vi "20T_Set_Setpoint.vi"(8 "error in (no error)":errorcluster, 10 "20T Control":T1={"Clamp"=TRUE, "Switch Heater"=TRUE, "Go to Zero"=TRUE, "Go to Set"=FALSE, "Go to Hold"=FALSE, "Setpoint (T)"=3.4572, "Rate (T/min)"=0.0, "Set Rate"=FALSE} {"Rate (T/min)" format="%6_5f"; "Setpoint (T)" format="%#4_5f"}, 11 "Mercury Reference In":T2) -> (0 "error out":errorcluster)   [LabVIEW 2016]
uses:
  Equipment/Mercury iXX/Public/Controls/Mercury Reference.ctl
  Equipment/Mercury iXX/Public/Controls/Comms Transport Layer.ctl
  Equipment/Mercury iXX/Private/Controls/Query Dynamic Reference.ctl
  Utility/Monitor Communication/Gustav/20T_Control.ctl
  Equipment/Mercury iXX/Public/Libraries/Magnet/Open/Open Magnet Device.vi
  Equipment/Mercury iXX/Mercury iXX.lvlib
  Equipment/Mercury iXX/Public/Libraries/Magnet.lvlib
panel:
  # "20 T"
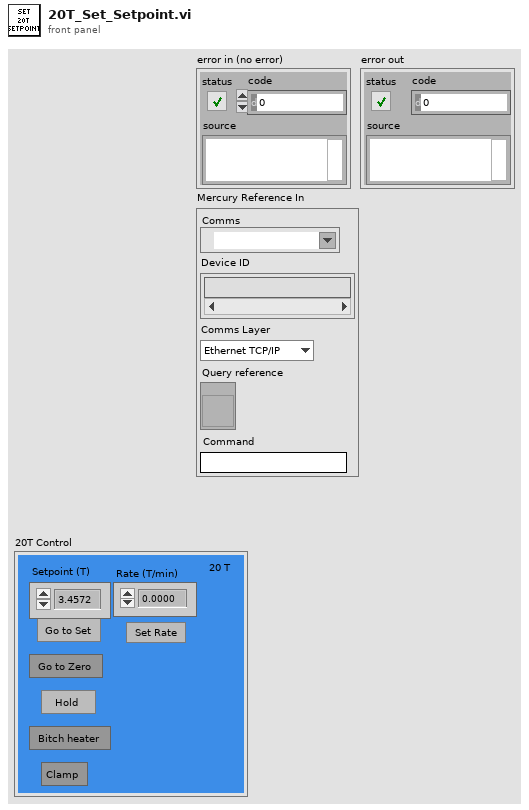
[diagram p1: front panel]
types:
  T1 = typedef "20T_Control.ctl" = cluster{"Clamp":bool, "Switch Heater":bool, "Go to Zero":bool, "Go to Set":bool, "Go to Hold":bool, "Setpoint (T)":dbl, "Rate (T/min)":dbl, "Set Rate":bool}
  T2 = typedef "Mercury iXX.lvlib/Mercury Reference.ctl" = cluster{"Comms":refnum<visa-resource-name>, "Device ID":string[], "Comms Layer":T3, "Command":string, "Query reference":T4}
  T3 = typedef "Mercury iXX.lvlib/Comms Transport Layer.ctl" = enum16{"Ethernet TCP/IP", "USB", "ISOBus - RS-232", "GPIB"}
  T4 = typedef "Mercury iXX.lvlib/Query Dynamic Reference.ctl" = refnum<vi>
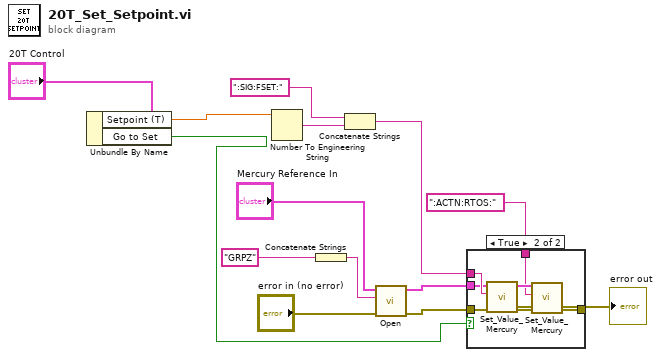
[diagram p0: block diagram]
diagram:
  n1 = Unbundle By Name("20T Control") -> ("Setpoint (T)"=w10:dbl, "Go to Set"=w2:bool)
  n2 = Number To Engineering String(4:w10) -> (0:w11:string)  [unwired: 3 in]
  n3 = Concatenate Strings("GRPZ" ("Device Identifier")) -> (w8:string)
  n4 = Concatenate Strings(":SIG:FSET:", w11) -> (w7:string)
  n5 = call-poly "Open.vi"("error in (no error)"="error in (no error)", "Device Identifier"=w8, "Mercury Reference In"="Mercury Reference In") -> ("error out"=w12:errorcluster, "Mercury Reference Out"=w13:T2)  [unwired: 1 in, 6 out]
  n6 = case shown="True" w2 {
    tunnel: w13 -> [_ w17]
    tunnel: w12 -> [w15 w20]
    tunnel: [w15 w18] -> w5
    tunnel: w7 -> [_ w21]
    tunnel: ":ACTN:RTOS:" -> [_ w16]
    frame False {
    }
    frame True {
      n7 = call "Set_Value_Mercury.vi"("error in"=w20, "Noun(s)"=w21, "Mercury Reference In"=w17) -> ("error out"=w19:errorcluster)  [unwired: 7 in, 1 out]
      n8 = call "Set_Value_Mercury.vi"("error in"=w19, "Noun(s)"=w16, "Mercury Reference In"=w17) -> ("error out"=w18:errorcluster)  [unwired: 7 in, 1 out]
    }
  }
  "error out" <- w5
